vi "Add.vi"() -> ()   [LabVIEW 2016]
panel:
  out "x+y":dbl
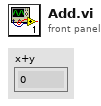
[diagram p1: front panel]
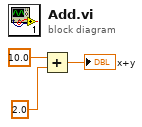
[diagram p0: block diagram]
diagram:
  n1 = Add(x=10.0, y=2.0) -> (x+y=→"x+y":dbl)
